vi "SCM Global.vi"() -> ()   [LabVIEW 2010]
panel:
  out "Channel List":T1(array[cluster])=[{"Board"=1, "Channel"=0, "Range"=1, "Interval"=1, "Offset"=0.0, "Multiplier"=20.0, "Field"="none", "Name"="QMeter 1 Temp"}, {"Board"=1, "Channel"=1, "Range"=1, "Interval"=1, "Offset"=0.0, "Multiplier"=20.0, "Field"="none", "Name"="QMeter 2 Temp"}, {"Board"=1, "Channel"=2, "Range"=1, "Interval"=1, "Offset"=0.0, "Multiplier"=20.0, "Field"="none", "Name"="QMeter 3 Temp"}, {"Board"=1, "Channel"=3, "Range"=1, "Interval"=1, "Offset"=0.0, "Multiplier"=20.0, "Field"="none", "Name"="QMeter 4 Temp"}, {"Board"=1, "Channel"=4, "Range"=1, "Interval"=1, "Offset"=0.0, "Multiplier"=10.0, "Field"="SepFlow", "Name"="Separator Flow"}, {"Board"=1, "Channel"=5, "Range"=1, "Interval"=1, "Offset"=0.0, "Multiplier"=10.0, "Field"="MainFlow", "Name"="Main Flow"}, {"Board"=1, "Channel"=6, "Range"=1, "Interval"=1, "Offset"=0.0, "Multiplier"=1.0, "Field"="HeliumVP", "Name"="HeliumVP"}, {"Board"=1, "Channel"=7, "Range"=5, "Interval"=1, "Offset"=0.0, "Multiplier"=100.0, "Field"="MagLevel", "Name"="Magnet Helium Level"}, {"Board"=1, "Channel"=8, "Range"=1, "Interval"=1, "Offset"=0.0, "Multiplier"=10.0, "Field"="RFVolts", "Name"="RF Voltmeter"}, {"Board"=1, "Channel"=9, "Range"=1, "Interval"=1, "Offset"=0.0, "Multiplier"=1.0, "Field"="uWavePower", "Name"="Microwave Power"}, {"Board"=1, "Channel"=10, "Range"=1, "Interval"=1, "Offset"=100.0, "Multiplier"=-200.0, "Field"="LN2Level", "Name"="Nitrogen Level"}, {"Board"=1, "Channel"=11, "Range"=1, "Interval"=1, "Offset"=-11.0, "Multiplier"=1.0, "Field"="VacPress", "Name"="Isolation Vacuum Pressure"}, {"Board"=1, "Channel"=12, "Range"=1, "Interval"=1, "Offset"=0.0, "Multiplier"=10.0, "Field"="Collector", "Name"="Collector Temperature"}] {"Offset" format="%.2f"; "Multiplier" format="%.2f"}
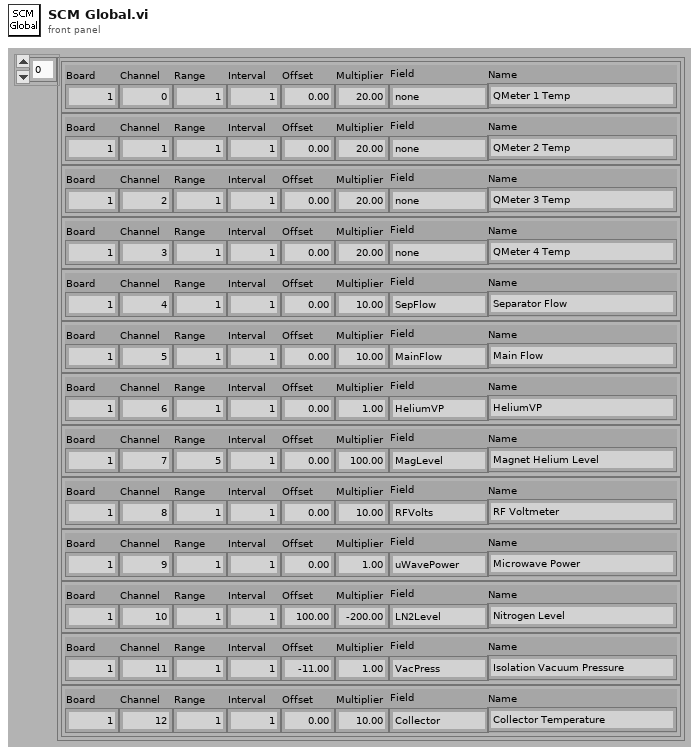
[diagram p1: front panel]
types:
  T1 = cluster{"Board":i32, "Channel":i32, "Range":i32, "Interval":i32, "Offset":dbl, "Multiplier":dbl, "Field":string, "Name":string}[]
diagram:
